vi "process_pixel_mapper.vi"() -> ()   [LabVIEW 2011, in "Fiberscope_library.lvlib"]
uses:
  Fiberscope_library.lvlib
  typedefs/pixel_per_spiral_I32.ctl
  typedefs/image_size_I32.ctl
  typedefs/element_streams_cluster.ctl
  typedefs/element_images_cluster.ctl
  typedefs/control_process_state_cluster.ctl
  typedefs/control_process_state_enum.ctl
  typedefs/feedback_to_watchdog.ctl
  typedefs/feedback_from_process_enum.ctl
  typedefs/all_scan_parameters_cluster.ctl
  typedefs/fiber_parameters_cluster.ctl
  typedefs/spiral_parameters_cluster.ctl
  typedefs/run_parameters_cluster.ctl
  typedefs/run_mode_enum.ctl
  typedefs/acquisition_parameters_cluster.ctl
  typedefs/smooth_coeffs_cluster.ctl
  typedefs/storage_parameters_cluster.ctl
  typedefs/mapping_corrections_cluster.ctl
  typedefs/pockels_corrections_cluster.ctl
panel:
  out "Phase corrections":dbl[][](graph)
  out "Amplitude corrections":dbl[][](graph)
  out "Local_exit":bool
  out "Pixelhits":dbl[][](graph)
  out "Pixel map":cluster{i32[], i32[]}(graph)
  out "error out":errorcluster
  in  "error in":errorcluster
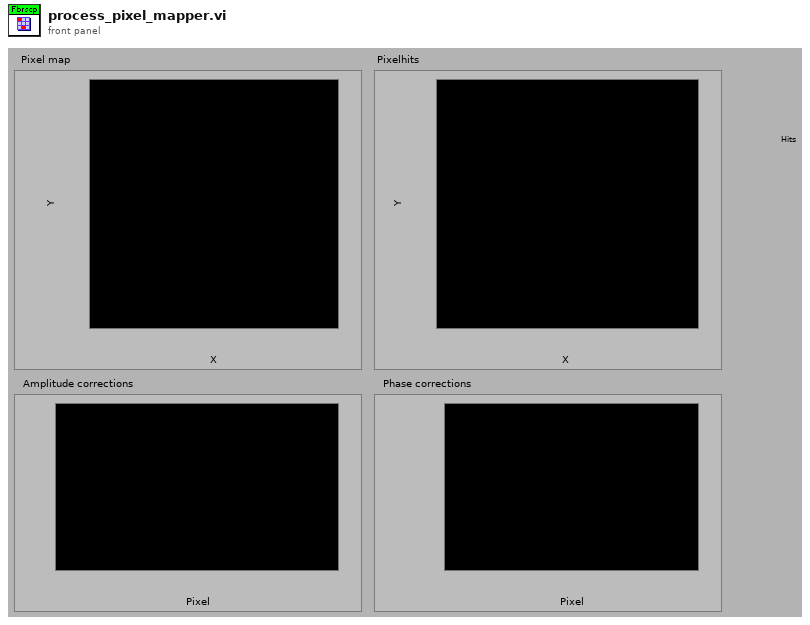
[diagram p1: front panel]
types:
  T1 = typedef "Fiberscope_library.lvlib/feedback_to_watchdog.ctl" = cluster{"Feedback_from_process_enum":T2, "Process_name":string}
  T2 = typedef "Fiberscope_library.lvlib/feedback_from_process_enum.ctl" = enum16{"Has_initialised", "Changed_parameters", "Has_started", "Has_stopped", "Has_quitted", "Is_running", "Has_finished", "Custom"}
  T3 = typedef "Fiberscope_library.lvlib/control_process_state_cluster.ctl" = cluster{"Control_process_state_enum":T4, "variant":variant}
  T4 = typedef "Fiberscope_library.lvlib/control_process_state_enum.ctl" = enum16{"Init", "Quit", "Start", "Stop", "Change_parameters", "Running", "Finish", "Custom"}
  T5 = typedef "Fiberscope_library.lvlib/element_streams_cluster.ctl" = cluster{"Streams_array":dbl[][], "#channels":i32, "Last element?":bool, "Forth (1) or back (0)?":bool}
  T6 = typedef "Fiberscope_library.lvlib/image_size_I32.ctl" = i32
  T7 = typedef "Fiberscope_library.lvlib/pixel_per_spiral_I32.ctl" = i32
  T8 = typedef "Fiberscope_library.lvlib/element_images_cluster.ctl" = cluster{"Images_array":dbl[][][], "#channels":i32, "Last element?":bool}
  T9 = typedef "Fiberscope_library.lvlib/all_scan_parameters_cluster.ctl" = cluster{"Fiber parameters":T10, "Spiral parameters":T11, "Run parameters":T12, "Acquisition parameters":T14, "Fiber parameters pixel_mapper":T10, "Smooth_coeffs_cluster":T15, "Storage parameters":T16, "Mapping corrections":T17, "Pockels corrections":T18}
  T10 = typedef "Fiberscope_library.lvlib/fiber_parameters_cluster.ctl" = cluster{"Frequency":dbl, "Amplitude X":dbl, "Amplitude Y":dbl, "Initial Amplitude X":dbl, "Initial Amplitude Y":dbl, "Phase":dbl}
  T11 = typedef "Fiberscope_library.lvlib/spiral_parameters_cluster.ctl" = cluster{"Imaging periods":dbl, "Settling periods":dbl, "Resting periods":dbl}
  T12 = typedef "Fiberscope_library.lvlib/run_parameters_cluster.ctl" = cluster{"Run mode":T13, "Averages per frame":u8, "No. of frames":u32}
  T13 = typedef "Fiberscope_library.lvlib/run_mode_enum.ctl" = enum16{"Continuous", "Single frame", "No. of frames"}
  T14 = typedef "Fiberscope_library.lvlib/acquisition_parameters_cluster.ctl" = cluster{"Cycles per pixel":u32, "Image size":T6, "Bidirectional acquisition":bool}
  T15 = typedef "Fiberscope_library.lvlib/smooth_coeffs_cluster.ctl" = cluster{"Coeff 1":dbl, "Coeff 2":dbl}
  T16 = typedef "Fiberscope_library.lvlib/storage_parameters_cluster.ctl" = cluster{"Autosave":bool, "Path":path}
  T17 = typedef "Fiberscope_library.lvlib/mapping_corrections_cluster.ctl" = cluster{"Phase increase":dbl, "Amplitude correction":dbl}
  T18 = typedef "Fiberscope_library.lvlib/pockels_corrections_cluster.ctl" = cluster{"Delay pixels":i32}
  T19 = typedef "Fiberscope_library.lvlib/lookup_arrays_ref_cluster.ctl" = cluster{"rows":refnum<data-value>, "cols":refnum<data-value>}
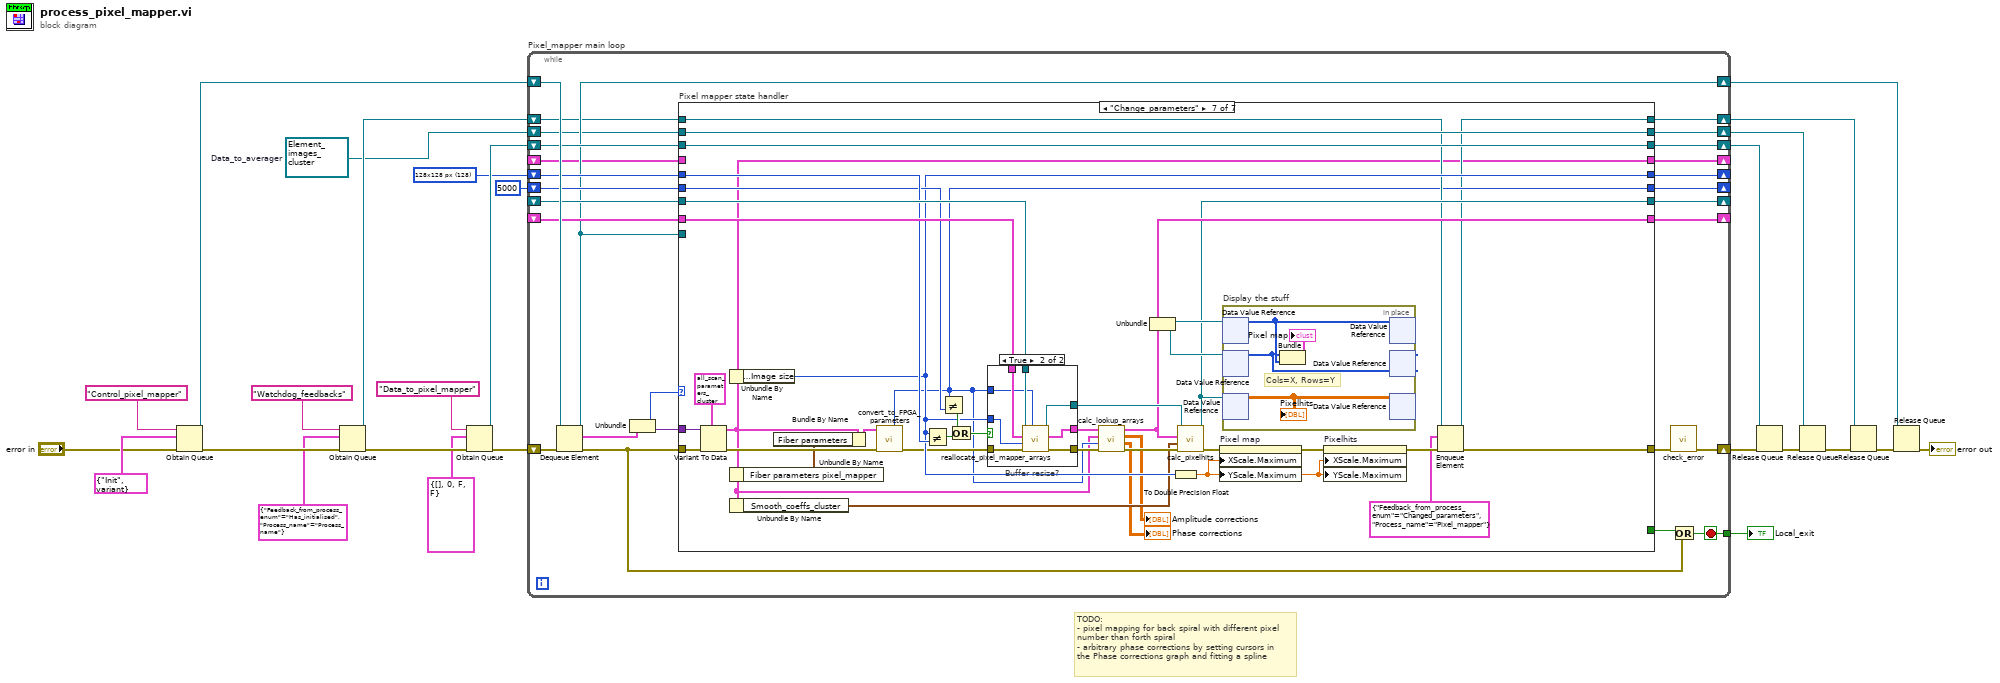
[diagram p0: block diagram]
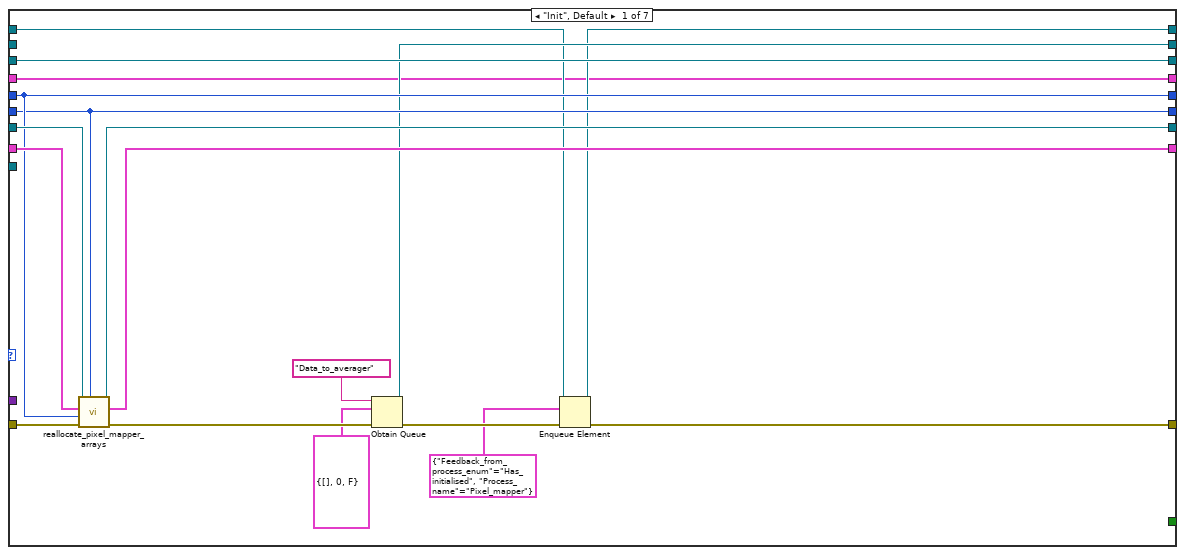
[diagram p2: hidden frame]
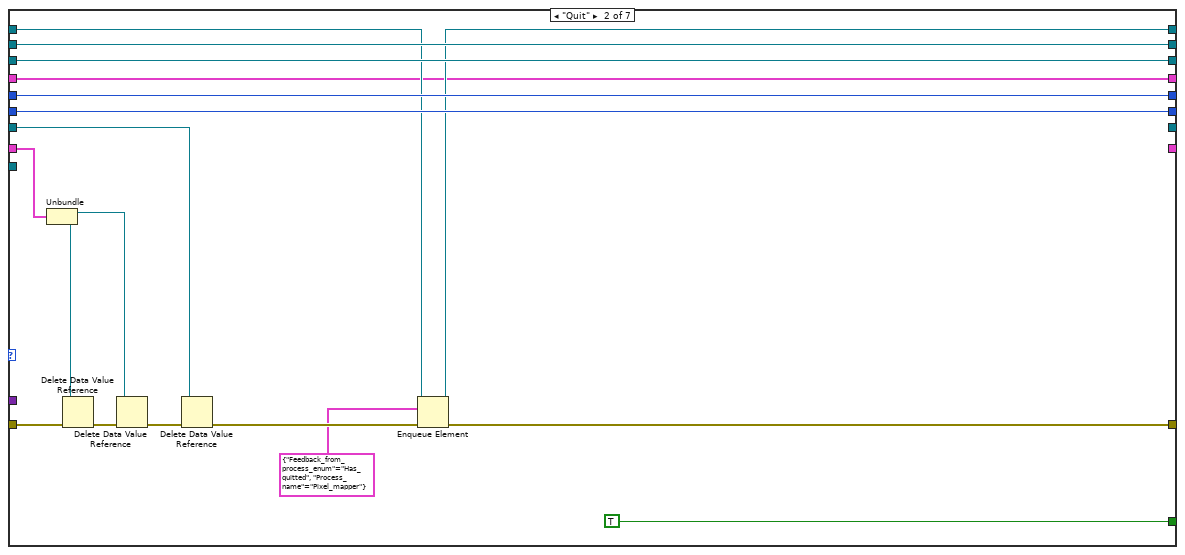
[diagram p3: hidden frame]
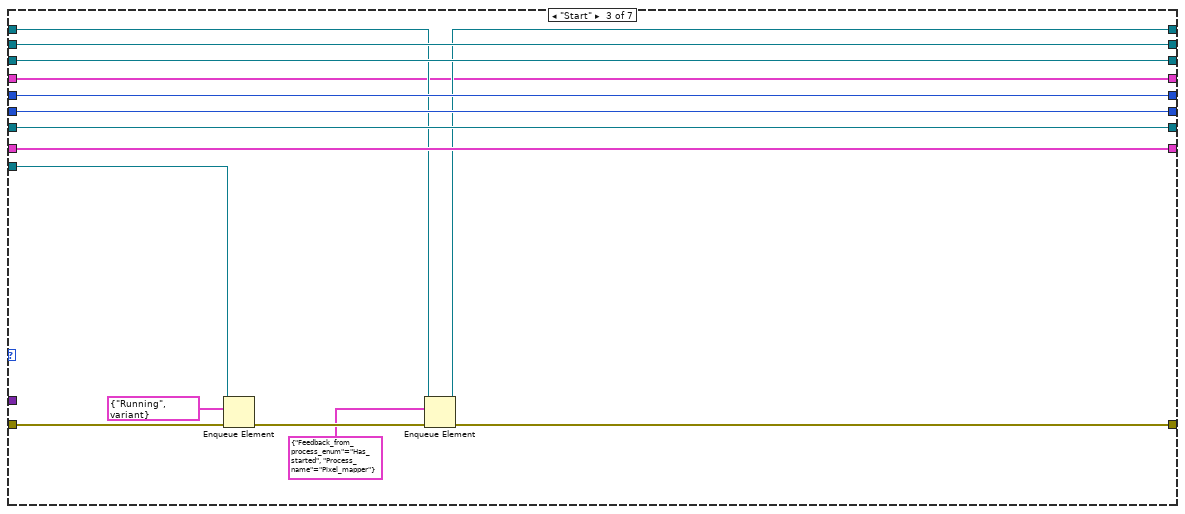
[diagram p4: hidden frame]
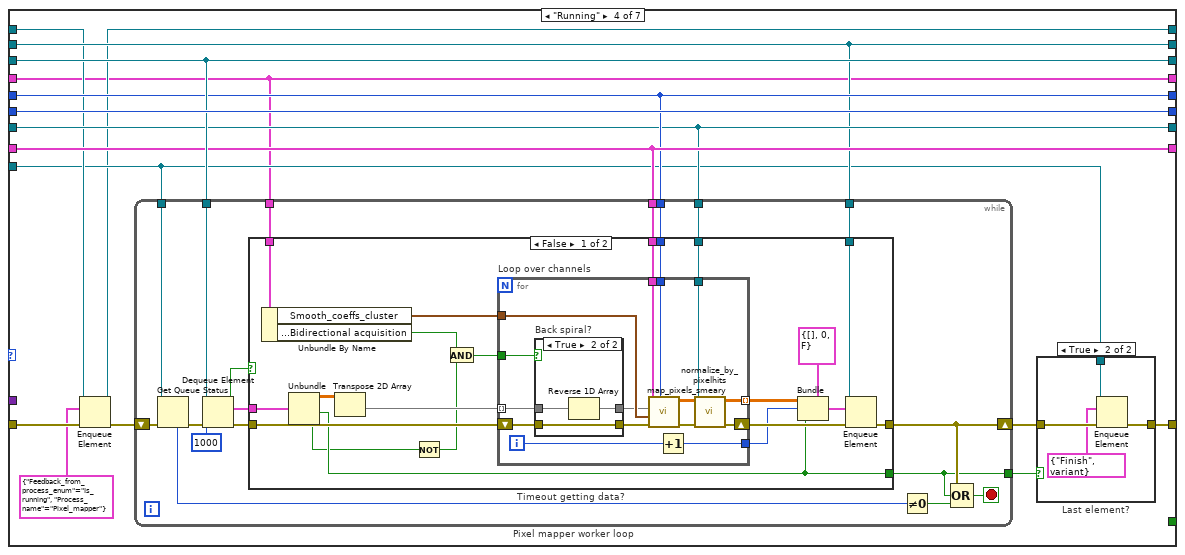
[diagram p5: hidden frame]
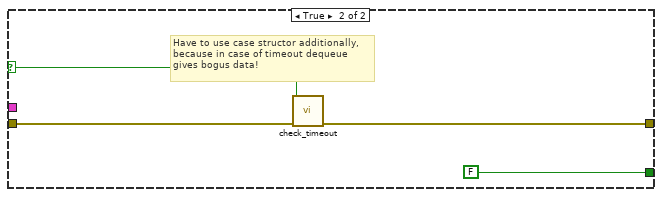
[diagram p8: hidden frame]
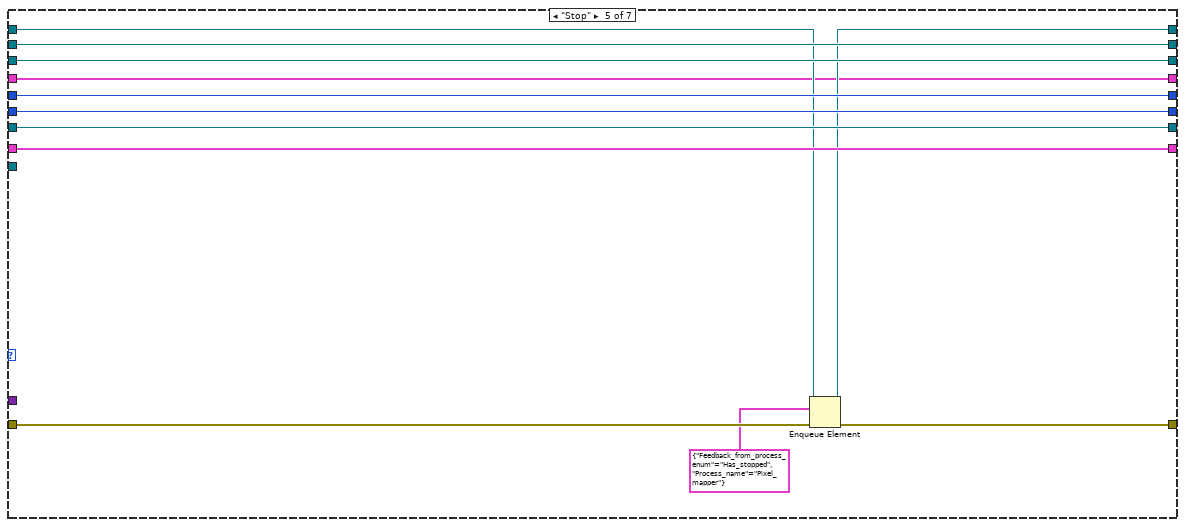
[diagram p9: hidden frame]
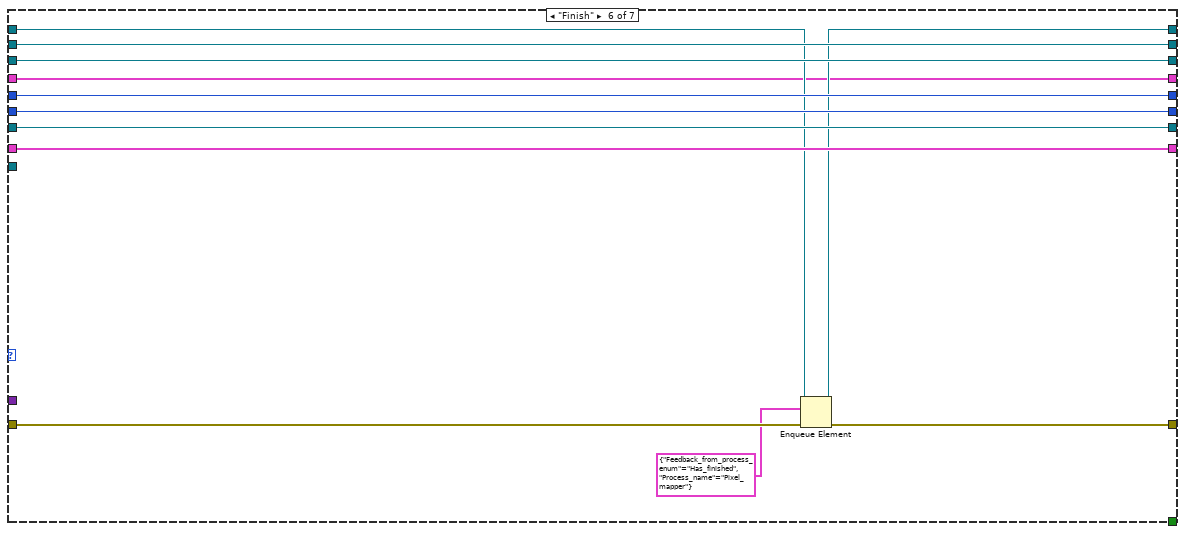
[diagram p10: hidden frame]
diagram:
  w6 = refnum<queue> refnum  # Data_to_averager
  w17 = T6 128 items=["128x128 px"=128, "256x256 px"=256, "512x512 px"=512] ("Image size")
  # "TODO:\n- pixel mapping for back spiral with different pixel\nnumber than forth spiral\n- arbitrary phase corrections by setting cursors in \nthe Phase corrections graph and fitting a spline"
  n1 = Obtain Queue(name (unnamed)="Control_pixel_mapper", element data type=T3 {"Control_process_state_enum"=enum."Init", "variant"=variant} ("Control_process_state_cluster"), error in (no error)="error in") -> (queue out=w1:refnum<queue>, error out=w16:errorcluster)  [unwired: 2 in, 1 out]
  n2 = Obtain Queue(name (unnamed)="Watchdog_feedbacks", element data type=T1 {"Feedback_from_process_enum"=enum."Has_initialised", "Process_name"="Process_name"}, error in (no error)=w16) -> (queue out=w13:refnum<queue>, error out=w15:errorcluster)  [unwired: 2 in, 1 out]
  n3 = Obtain Queue(name (unnamed)="Data_to_pixel_mapper", element data type=T5 {"Streams_array"=[], "#channels"=0, "Last element?"=FALSE, "Forth (1) or back (0)?"=FALSE} ("Element_from_DAQ_cluster"), error in (no error)=w15) -> (queue out=w21:refnum<queue>, error out=w23:errorcluster)  [unwired: 2 in, 1 out]
  n4 = while "Pixel_mapper main loop" {
    shift-right: [w47] -> w20
    shift-left: w23 -> [w53]
    shift-right: [w39] -> _
    shift-left: w17 -> [w44]
    shift-right: [w43] -> _
    shift-left: _ -> [w42]
    shift-right: [w41] -> _
    shift-left: _ -> [w40]
    shift-right: [w37] -> _
    shift-left: T7 5000 ("Pixels per spiral") -> [w38]
    shift-right: [w34] -> w8
    shift-left: w6 -> [w35]
    shift-right: [w36] -> w24
    shift-left: w1 -> [w52]
    shift-right: [w45] -> w19
    shift-left: w21 -> [w46]
    shift-right: [w32] -> w11
    shift-left: w13 -> [w33]
    tunnel: [w29] -> w2
    shift-right: [w28] -> _
    shift-left: _ -> [w27]
    stop <- w29 stop-if-true
    n5 = Dequeue Element(queue=w52, error in (no error)=w53) -> (queue out=w36:refnum<queue>, element=w51:T3, error out=w30:errorcluster)  [unwired: 1 in, 1 out]
    n6 = Unbundle(w51) -> ("Control_process_state_enum"=w49:T4, "variant"=w50:variant)
    n7 = case "Pixel mapper state handler" shown="\"Change_parameters\"" w49 {
      tunnel: w30 -> [w70 w86 w96 w114 w194 w206 w249]
      tunnel: [w59 w76 w94 w110 w193 w205 w226] -> w48
      tunnel: w50 -> [_ _ _ _ _ _ w248]
      tunnel: w46 -> [w71 w89 w103 w119 w200 w212 w250]
      tunnel: [w71 w89 w103 w119 w200 w212 w250] -> w45
      tunnel: w44 -> [w65 w88 w101 w117 w197 w209 w236]
      tunnel: [w66 _ w100 w116 w199 w211 w237] -> w43
      tunnel: w42 -> [w68 w82 w100 w116 w199 w211 w244]
      tunnel: [w67 _ w102 w118 w198 w210 w240] -> w41
      tunnel: w40 -> [w69 w87 w102 w118 w198 w210 w245]
      tunnel: [w65 w88 w101 w117 w197 w209 w228] -> w39
      tunnel: w38 -> [w62 w80 w104 w120 w196 w208 w232]
      tunnel: [w62 w80 w104 w120 w196 w208 w221] -> w37
      tunnel: w36 -> [_ _ w97 w108 _ _ _]
      tunnel: w35 -> [_ w79 w99 w115 w195 w207 w241]
      tunnel: [_ TRUE _ _ _ _ _] -> w31
      tunnel: [w61 w79 w99 w115 w195 w207 w241] -> w34
      tunnel: w33 -> [w58 w75 w98 w112 w192 w204 w225]
      tunnel: [w56 w74 w92 w107 w191 w203 w220] -> w32
      tunnel: [w54 w72 w90 w105 w189 w201 w217] -> w28
      tunnel: w27 -> [w54 w72 w90 w105 w189 w201 _]
      frame "Init", Default {
        n8 = call "reallocate_pixel_mapper_arrays.vi"("New pixels per spiral"=w62, "error in"=w70, "New image size"=w65, "Lookup arrays in"=w69, "Pixelhits array in"=w68) -> ("error out"=w64:errorcluster, "Lookup arrays out"=w67:T19, "Pixelhits array out"=w66:refnum<data-value>)  [unwired: 4 in]
        n9 = Obtain Queue(name (unnamed)="Data_to_averager", element data type=T8 {"Images_array"=[], "#channels"=0, "Last element?"=FALSE} ("Element_images_cluster"), error in (no error)=w64) -> (queue out=w61:refnum<queue>, error out=w60:errorcluster)  [unwired: 2 in, 1 out]
        n10 = Enqueue Element(queue=w58, element=T1 {"Feedback_from_process_enum"=enum."Has_initialised", "Process_name"="Pixel_mapper"}, error in (no error)=w60) -> (queue out=w56:refnum<queue>, error out=w59:errorcluster)  [unwired: 1 in, 1 out]
      }
      frame "Quit" {
        n11 = Unbundle(w87) -> ("rows"=w83:refnum<data-value>, "cols"=w85:refnum<data-value>)
        n12 = Delete Data Value Reference(data value reference=w85, error in=w86) -> (error out=w84:errorcluster)  [unwired: 1 out]
        n13 = Delete Data Value Reference(data value reference=w83, error in=w84) -> (error out=w81:errorcluster)  [unwired: 1 out]
        n14 = Delete Data Value Reference(data value reference=w82, error in=w81) -> (error out=w77:errorcluster)  [unwired: 1 out]
        n15 = Enqueue Element(queue=w75, element=T1 {"Feedback_from_process_enum"=enum."Has_quitted", "Process_name"="Pixel_mapper"}, error in (no error)=w77) -> (queue out=w74:refnum<queue>, error out=w76:errorcluster)  [unwired: 1 in, 1 out]
      }
      frame "Start" {
        n16 = Enqueue Element(queue=w97, element=T3 {"Control_process_state_enum"=enum."Running", "variant"=variant} ("Control_process_state_cluster"), error in (no error)=w96) -> (error out=w95:errorcluster)  [unwired: 1 in, 2 out]
        n17 = Enqueue Element(queue=w98, element=T1 {"Feedback_from_process_enum"=enum."Has_started", "Process_name"="Pixel_mapper"}, error in (no error)=w95) -> (queue out=w92:refnum<queue>, error out=w94:errorcluster)  [unwired: 1 in, 1 out]
      }
      frame "Running" {
        n18 = Enqueue Element(queue=w112, element=T1 {"Feedback_from_process_enum"=enum."Is_running", "Process_name"="Pixel_mapper"}, error in (no error)=w114) -> (queue out=w107:refnum<queue>, error out=w113:errorcluster)  [unwired: 1 in, 1 out]
        n19 = while "Pixel mapper worker loop" {
          shift-right: [w130] -> w111
          shift-left: w113 -> [w138]
          tunnel: w119 -> [w143]
          tunnel: w108 -> [w139]
          tunnel: w115 -> [w136]
          tunnel: w118 -> [w133]
          tunnel: w117 -> [w132]
          tunnel: w116 -> [w131]
          tunnel: [w127] -> w109
          tunnel: w105 -> [w126]
          stop <- w140 stop-if-true
          n20 = Get Queue Status(queue=w139, error in (no error)=w138) -> (error out=w137:errorcluster, # elements in queue=w142:i32)  [unwired: 1 in, 6 out]
          n21 = Dequeue Element(queue=w143, timeout in ms (-1)=1000, error in (no error)=w137) -> (element=w128:T5, timed out?=w134:bool, error out=w129:errorcluster)  [unwired: 1 out]
          n22 = case "Timeout getting data?" shown="False" w134 {
            selector: w134 -> [_ w186]
            tunnel: w129 -> [w162 w188]
            tunnel: [w164 w187] -> w130
            tunnel: w136 -> [w163 _]
            tunnel: w128 -> [w152 _]
            tunnel: w133 -> [w161 _]
            tunnel: w132 -> [w160 _]
            tunnel: w131 -> [w158 _]
            tunnel: [w150 FALSE ("Last element?")] -> w127
            tunnel: w126 -> [w149 _]
            frame False {
              n23 = Unbundle By Name(w149) -> ("Smooth_coeffs_cluster"=w148:T15, "Acquisition parameters.Bidirectional acquisition"=w145:bool)
              n24 = Unbundle(w152) -> ("Streams_array"=w153:dbl[][], "Last element?"=w150:bool, "Forth (1) or back (0)?"=w146:bool)  [unwired: 1 out]
              n25 = Transpose 2D Array(2D array=w153) -> (transposed array=w151:dbl[][])
              n26 = Not(x=w146) -> (.not. x?=w147:bool)
              n27 = And(x=w145, y=w147) -> (x .and. y?=w144:bool)
              n28 = for "Loop over channels" {
                tunnel: w151 -> [w167] mode=indexing
                tunnel: w161 -> [w179]
                tunnel: w160 -> [w178]
                shift-right: [w176] -> w159
                shift-left: w162 -> [w169]
                tunnel: [w174] -> w155 mode=indexing
                tunnel: w158 -> [w173]
                tunnel: [w171] -> w154
                tunnel: w148 -> [w170]
                tunnel: w144 -> [w165]
                i -> [w172]
                n29 = case "Back spiral?" shown="True" w165 {
                  tunnel: w169 -> [w180 w184]
                  tunnel: [w180 w184] -> w168
                  tunnel: w167 -> [w181 w183]
                  tunnel: [w181 w182] -> w166
                  frame False {
                  }
                  frame True {
                    n30 = Reverse 1D Array(array=w183) -> (reversed array=w182:dbl[])
                  }
                }
                n31 = call "map_pixels_smeary.vi"("Image size"=w178, "error in"=w168, "Smooth_coeffs_cluster"=w170, "Stream in"=w166, "Lookup arrays"=w179) -> ("error out"=w177:errorcluster, "Image out"=w175:dbl[][])  [unwired: 5 in]
                n32 = Increment(x=w172) -> (x+1=w171:i32)
                n33 = call "normalize_by_pixelhits.vi"("error in"=w177, "Pixelhits array"=w173, "Image in"=w175) -> ("error out"=w176:errorcluster, "Image out"=w174:dbl[][])  [unwired: 7 in]
              }
              n34 = Bundle(cluster=T8 {"Images_array"=[], "#channels"=0, "Last element?"=FALSE} ("Element_images_cluster"), "Images_array"=w155, "#channels"=w154, "Last element?"=w150) -> (w156:T8)
              n35 = Enqueue Element(queue=w163, element=w156, error in (no error)=w159) -> (error out=w164:errorcluster)  [unwired: 1 in, 2 out]
            }
            frame True {
              # "Have to use case structor additionally,\nbecause in case of timeout dequeue\ngives bogus data!"
              n36 = call "check_timeout.vi"("error in"=w188, "Timeout?"=w186) -> ("error out"=w187:errorcluster)  [unwired: 9 in]
            }
          }
          n37 = Not Equal To 0?(x=w142) -> (x != 0?=w141:bool)
          n38 = Compound Arithmetic op=OR(w130, w127, w141) -> (w140:bool)
        }
        n39 = case "Last element?" shown="True" w109 {
          tunnel: w111 -> [w121 w125]
          tunnel: [w121 w124] -> w110
          tunnel: w108 -> [_ w123]
          frame False {
          }
          frame True {
            n40 = Enqueue Element(queue=w123, element=T3 {"Control_process_state_enum"=enum."Finish", "variant"=variant} ("Control_process_state_cluster"), error in (no error)=w125) -> (error out=w124:errorcluster)  [unwired: 1 in, 2 out]
          }
        }
      }
      frame "Stop" {
        n41 = Enqueue Element(queue=w192, element=T1 {"Feedback_from_process_enum"=enum."Has_stopped", "Process_name"="Pixel_mapper"}, error in (no error)=w194) -> (queue out=w191:refnum<queue>, error out=w193:errorcluster)  [unwired: 1 in, 1 out]
      }
      frame "Finish" {
        n42 = Enqueue Element(queue=w204, element=T1 {"Feedback_from_process_enum"=enum."Has_finished", "Process_name"="Pixel_mapper"}, error in (no error)=w206) -> (queue out=w203:refnum<queue>, error out=w205:errorcluster)  [unwired: 1 in, 1 out]
      }
      frame "Change_parameters" {
        n43 = Variant To Data(error in=w249, type=T9 {"Fiber parameters"={"Frequency"=100.0, "Amplitude X"=0.0, "Amplitude Y"=0.0, "Initial Amplitude X"=0.0, "Initial Amplitude Y"=0.0, "Phase"=0.0}, "Spiral parameters"={"Imaging periods"=1.0, "Settling periods"=1.0, "Resting periods"=1.0}, "Run parameters"={"Run mode"=enum."Continuous", "Averages per frame"=0, "No. of frames"=0}, "Acquisition parameters"={"Cycles per pixel"=0, "Image size"=1, "Bidirectional acquisition"=FALSE}, "Fiber parameters pixel_mapper"={"Frequency"=0.0, "Amplitude X"=0.0, "Amplitude Y"=0.0, "Initial Amplitude X"=0.0, "Initial Amplitude Y"=0.0, "Phase"=0.0}, "Smooth_coeffs_cluster"={"Coeff 1"=0.0, "Coeff 2"=0.0}, "Storage parameters"={"Autosave"=FALSE, "Path"=path ""}, "Mapping corrections"={"Phase increase"=0.0, "Amplitude correction"=0.0}, "Pockels corrections"={"Delay pixels"=0}} ("All scan parameters"), Variant=w248) -> (data=w217:T9, error out=w223:errorcluster)
        n44 = Unbundle By Name(w217) -> ("Acquisition parameters.Image size"=w228:T6)
        n45 = Unbundle By Name(w217) -> ("Fiber parameters pixel_mapper"=w215:T10)
        n46 = Unbundle By Name(w217) -> ("Smooth_coeffs_cluster"=w218:T15)
        n47 = Bundle By Name(cluster=w217, "Fiber parameters"=w215) -> (w216:T9)
        n48 = call "convert_to_FPGA_parameters.vi"("error in"=w223, "All scan parameters"=w216) -> ("error out"=w222:errorcluster, "Pixels per spiral"=w221:i32)  [unwired: 5 in, 3 out]
        n49 = Not Equal?(x=w228, y=w236) -> (x != y?=w234:bool)
        n50 = Not Equal?(x=w221, y=w232) -> (x != y?=w235:bool)
        n51 = Or(x=w235, y=w234) -> (x .or. y?=w233:bool)
        n52 = case "Buffer resize?" shown="True" w233 {
          tunnel: w222 -> [w257 w265]
          tunnel: [w257 w264] -> w246
          tunnel: w245 -> [w256 w262]
          tunnel: w244 -> [w255 w261]
          tunnel: [w256 w260] -> w243
          tunnel: [w255 w259] -> w242
          tunnel: w228 -> [_ w263]
          tunnel: w221 -> [_ w258]
          frame False {
          }
          frame True {
            n53 = call "reallocate_pixel_mapper_arrays.vi"("New pixels per spiral"=w258, "error in"=w265, "New image size"=w263, "Lookup arrays in"=w262, "Pixelhits array in"=w261) -> ("error out"=w264:errorcluster, "Lookup arrays out"=w260:T19, "Pixelhits array out"=w259:refnum<data-value>)  [unwired: 4 in]
          }
        }
        n54 = call "calc_lookup_arrays.vi"("error in"=w246, "Pixels per spiral"=w221, "All scan parameters"=w217, "Lookup arrays in"=w243) -> ("error out"=w247:errorcluster, "Phase corrections"=→"Phase corrections":dbl[][], "Amplitude corrections"=→"Amplitude corrections":dbl[][], "Lookup arrays out"=w240:T19)  [unwired: 4 in]
        n55 = Unbundle(w240) -> ("rows"=w239:refnum<data-value>, "cols"=w238:refnum<data-value>)
        n56 = To Double Precision Float(number=w228) -> (double precision float=w229:dbl)
        n57 = call "calc_pixelhits.vi"("error in"=w247, "Smooth_coeffs_cluster"=w218, "Lookup arrays"=w240, "Pixelhits array in"=w242) -> ("error out"=w231:errorcluster, "Pixelhits array out"=w237:refnum<data-value>)  [unwired: 6 in]
        n58 = property on="Pixel map" class="XYGraph (strict)"(error in=w231, "XScale.Maximum"=w229, "YScale.Maximum"=w229) -> (error out=w230:errorcluster)  [unwired: 1 in, 1 out]
        n59 = in-place "Display the stuff" {
          # "Cols=X, Rows=Y"
          n60 = in-place-dvr #1(w239) -> (w254:i32[])  [unwired: 1 out]
          n61 = in-place-dvr #2(w238) -> (w253:i32[])  [unwired: 1 out]
          n62 = in-place-dvr #3(w237) -> (w251:dbl[][])  [unwired: 1 out]
          "Pixelhits" <- w251
          n63 = Bundle(w253, w254) -> (→"Pixel map":cluster{i32[], i32[]})  [unwired: 1 in]
          n64 = in-place-dvr #1(w254) -> ()  [unwired: 2 out]
          n65 = in-place-dvr #2(w253) -> ()  [unwired: 2 out]
          n66 = in-place-dvr #3(w251) -> ()  [unwired: 2 out]
        }
        n67 = property on="Pixelhits" class="IntGraph (strict)"(error in=w230, "XScale.Maximum"=w229, "YScale.Maximum"=w229) -> (error out=w227:errorcluster)  [unwired: 1 in, 1 out]
        n68 = Enqueue Element(queue=w225, element=T1 {"Feedback_from_process_enum"=enum."Changed_parameters", "Process_name"="Pixel_mapper"}, error in (no error)=w227) -> (queue out=w220:refnum<queue>, error out=w226:errorcluster)  [unwired: 1 in, 1 out]
      }
    }
    n69 = call "check_error.vi"("error in"=w48) -> ("error out"=w47:errorcluster)  [unwired: 10 in]
    n70 = Or(x=w31, y=w30) -> (x .or. y?=w29:bool)
  }
  "Local_exit" <- w2
  n71 = Release Queue(queue=w19, error in (no error)=w20) -> (error out=w10:errorcluster)  [unwired: 1 in, 2 out]
  n72 = Release Queue(queue=w8, error in (no error)=w10) -> (error out=w9:errorcluster)  [unwired: 1 in, 2 out]
  n73 = Release Queue(queue=w11, error in (no error)=w9) -> (error out=w12:errorcluster)  [unwired: 1 in, 2 out]
  n74 = Release Queue(queue=w24, error in (no error)=w12) -> (error out=→"error out":errorcluster)  [unwired: 1 in, 2 out]
